vi "DSiam.vi"() -> ()   [LabVIEW 2011]
uses:
  SIAM/SIAM_command.ctl
  SIAM/SIAM-send.ctl
panel:
  out "PWD send":u32[](array[numeric])
  out "code":i32
  out "KEy":string
  out "notifier name":string
  out "send error":errorcluster
  out "value send":dbl
  out "Running":bool
  in  "Scales and Tickets":T1(array[cluster])=[{"ticketID"=514, "Queue/Variable"=FALSE, "name"="stage.z", "Scale"=2e-09, "Offset(HWunits)"=0.0}]
  out "address":string="10.153.70.38"
  out "remote port or service name":u16=3
  out "connect error":errorcluster
  out "Return":i32[](array[numeric]) format="%.0x"
  out "recieve error":errorcluster
  out "Connected":bool
  # "to do\nlimits?\nclosed loop über DSmartmove oder DSIAM oder Smartconnect?\n...\n...\n\n.. Objektivwechsel..."
  # "1122=normal exit"
  # "66=normal exit"
  # "bisher üblich steps/units!!! Logischer für filter!"
  # "becarefull with queues, if there is no reciever it is a memory leak"
  # "ticket  is also inside SIAM-TMSI.vi"
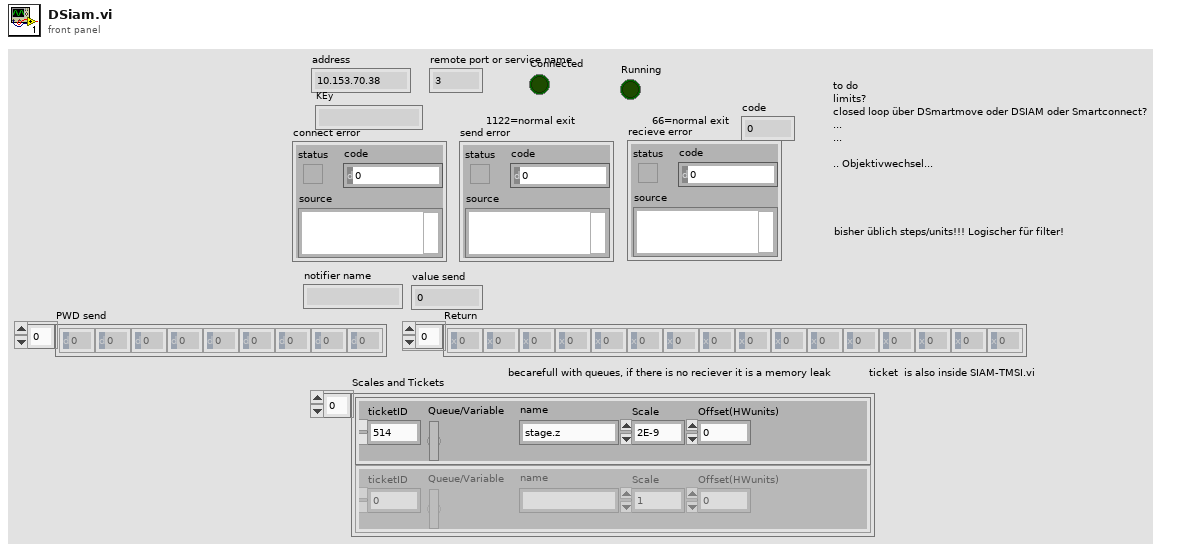
[diagram p1: front panel]
types:
  T1 = cluster{"ticketID":i32, "Queue/Variable":bool, "name":string, "Scale":dbl, "Offset(HWunits)":dbl}[]
  T2 = enum16{"None/#Datasets", "Clear", "TagValueOf#", "AddValues", "ReadValue", "ChangeValue", "Get all"}
  T3 = cluster{"Scale":dbl, "Offset(HWunits)":dbl, "ticketID":i32}[]
  T4 = typedef "SIAM-send.ctl" = enum16{"validID", "storeID", "enable", "rundirect", "sendlist", "run", "stop", "readRegister", "sendValue", "storeStatus"}
  T5 = enum8{"Ch0", "Ch1", "x-Galvo", "y-Galvo", "z-Focus"}
  T6 = enum16{"Ch0", "Ch1", "x-Galvo", "y-Galvo", "z-Focus"}
  T7 = enum16{"Standard", "Buffered", "CRLF", "Immediate"}
  T8 = typedef "SIAM_command.ctl" = u32
  T9 = cluster{"Delay 10µs":u32, "command":T8, "P0":i32, "P1":i32, "P2":i32, "P3":i32, "P4":i32, "P5-ticket":i32}
  T10 = cluster{"Scale":ext, "Offset(HWunits)":ext, "ticketID":i32}[]
  T11 = cluster{"ticketID":i32, "Queue/Variable":bool, "name":string, "Scale":dbl, "Offset(HWunits)":dbl}
  T12 = cluster{"variables":string[], cluster{"Scale":ext, "Offset(HWunits)":ext, "ticketID":i32}[]}
  T13 = cluster{"default value 2":dbl, "default value 1":dbl}
  T14 = cluster{"Delay 10µs":u32, "command":T8, "P0":i32, "P1":i32, "P2":i32, "P3":i32, "P4":i32, "P5-ticket":i32}[]
  T15 = cluster{"Scale":ext, "Offset(HWunits)":ext, "ticketID":i32}
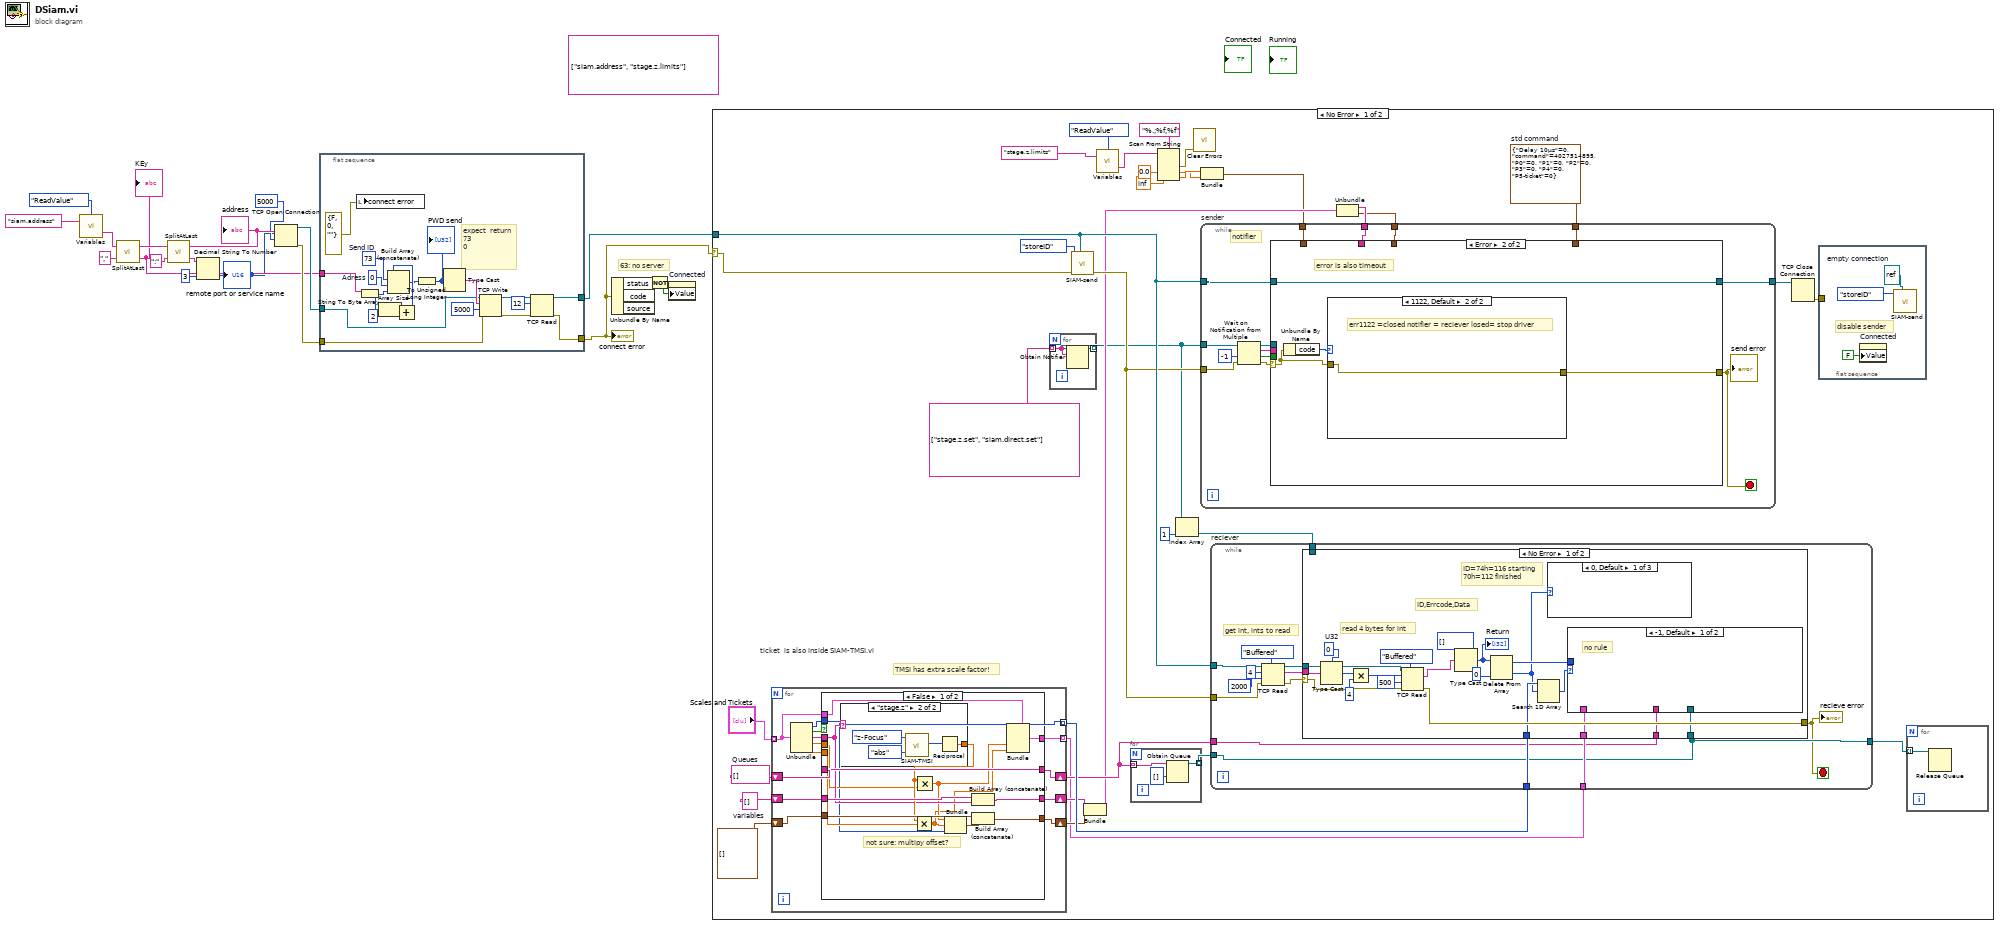
[diagram p0: block diagram]
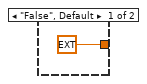
[diagram p2: hidden frame]
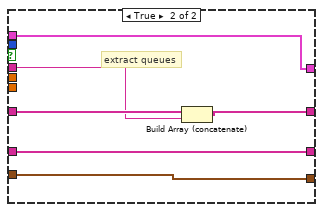
[diagram p3: hidden frame]
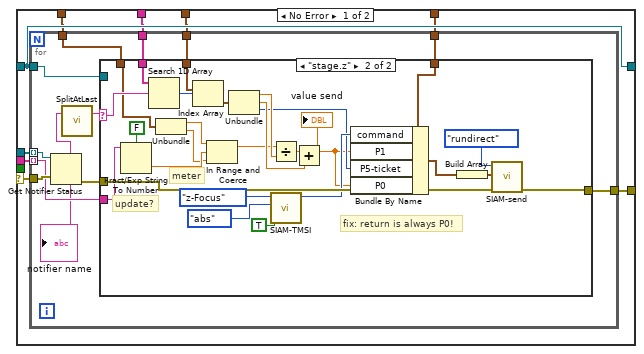
[diagram p4: hidden frame]
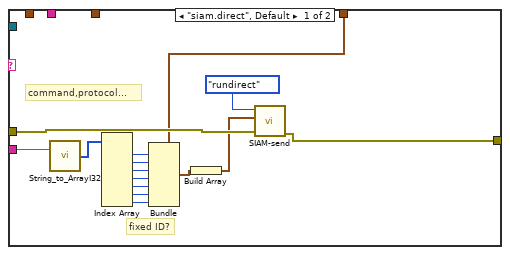
[diagram p5: hidden frame]
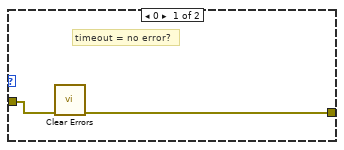
[diagram p6: hidden frame]
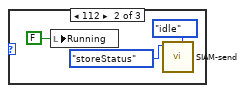
[diagram p7: hidden frame]
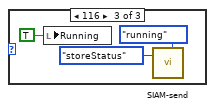
[diagram p8: hidden frame]
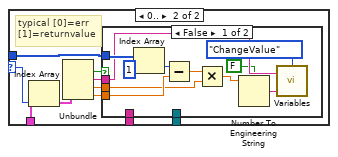
[diagram p9: hidden frame]
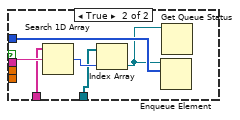
[diagram p10: hidden frame]
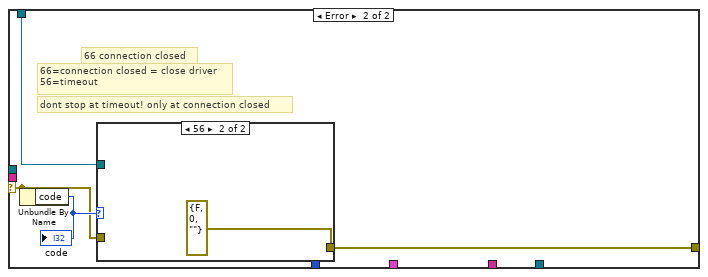
[diagram p11: hidden frame]
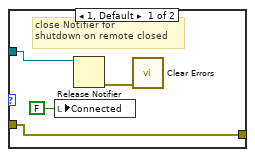
[diagram p12: hidden frame]
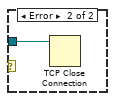
[diagram p13: hidden frame]
diagram:
  (unwired) string[] ["siam.address", "stage.z.limits"]
  # "63: no server"
  n1 = call "Variables.vi"("Tag in"="siam.address", "Command"=T2."ReadValue") -> ("value out"=w9:string)  [unwired: 2 in, 1 out]
  n2 = call "SplitAtLast.vi"("search char"=",", "In-String"=w9) -> ("end"=w4:string, "Front (default)"=w7:string)
  "KEy" <- w4
  n3 = call "SplitAtLast.vi"("search char"=":", "In-String"=w7) -> ("end"=w13:string, "Front (default)"=w14:string)
  "address" <- w14
  n4 = Decimal String To Number(string=w13, default (0L)=3 ("default (0 I32)")) -> (number=w3:i32)  [unwired: 1 in, 1 out]
  "remote port or service name" <- w3
  n5 = TCP Open Connection(address=w14, remote port or service name=w3, timeout ms (60000)=5000) -> (connection ID=w5:refnum<k5>, error out=w6:errorcluster)  [unwired: 1 in, 1 out]
  n6 = flat-sequence {
    tunnel: w5 -> [w33]
    tunnel: w6 -> [w32]
    tunnel: [w22] -> w1
    tunnel: [w24] -> w2
    tunnel: w4 -> [w19]
    frame #0 {
      w30 = 0  # Adress
      w34 = u8 73  # Send ID
      # "expect  return\n73\n0"
      n7 = local write "connect error"(errorcluster {"status"=FALSE, "code"=0, "source"=""} ("recieve error")) -> ()
      n8 = String To Byte Array(string=w19) -> (unsigned byte array=w29:u8[])
      n9 = Array Size(array=w29) -> (size(s)=w35:i32)
      n10 = Add(x=w35, y=2) -> (x+y=w27:i32)
      n11 = Build Array (concatenate)(w27, w34, w30, w29) -> (w26:i32[])
      n12 = To Unsigned Long Integer(number=w26) -> (unsigned 32bit integer=w36:u32[])
      "PWD send" <- w36
      n13 = Type Cast(x=w36) -> (*(type *) &x=w37:string)  [unwired: 1 in]
      n14 = TCP Write(connection ID=w33, data in=w37, error in (no error)=w32, 9:5000 ("timeout ms (25000)")) -> (connection ID out=w25:refnum<k5>, error out=w23:errorcluster)  [unwired: 1 out]
      n15 = TCP Read(connection ID=w25, bytes to read=12, error in (no error)=w23) -> (connection ID out=w24:refnum<k5>, error out=w22:errorcluster)  [unwired: 2 in, 1 out]
    }
  }
  n16 = Unbundle By Name(w1) -> ("status"=w18:bool)  [unwired: 2 out]
  n17 = Not(x=w18) -> (.not. x?=w11:bool)
  n18 = property on="Connected" class="Bool (strict)"("Value"=w11) -> ()  [unwired: 2 in, 2 out]
  n19 = case shown="No Error" w1 {
    selector: w1 -> [w41 _]
    tunnel: w2 -> [w65 w282]
    frame No Error {
      w61 = string[] []  # variables
      w62 = T9 {"Delay 10µs"=0, "command"=4027514895, "P0"=0, "P1"=0, "P2"=0, "P3"=0, "P4"=0, "P5-ticket"=0}  # std command
      w69 = string[] []  # Queues
      # "ticket  is also inside SIAM-TMSI.vi"
      # "TMSI has extra scale factor!"
      n20 = for {
        tunnel: "Scales and Tickets" -> [w86] mode=indexing
        tunnel: [w81] -> w71 mode=indexing
        shift-right: [w91] -> w66
        shift-left: w69 -> [w92]
        shift-right: [w89] -> w59
        shift-left: w61 -> [w90]
        shift-right: [w87] -> w58
        shift-left: T3 [] -> [w88]
        tunnel: [w80] -> w53 mode=indexing
        n21 = Unbundle(w86) -> ("ticketID"=w81:i32, "Queue/Variable"=w85:bool, "name"=w84:string, "Scale"=w83:dbl, "Offset(HWunits)"=w82:dbl)
        n22 = case shown="False" w85 {
          tunnel: w92 -> [w107 w118]
          tunnel: [w107 w116] -> w91
          tunnel: w84 -> [w100 w117]
          tunnel: w86 -> [w96 w113]
          tunnel: w90 -> [w106 w115]
          tunnel: [w105 w115] -> w89
          tunnel: w88 -> [w104 w114]
          tunnel: [w103 w114] -> w87
          tunnel: w83 -> [w98 _]
          tunnel: w82 -> [w99 _]
          tunnel: w81 -> [w97 _]
          tunnel: [w93 w113] -> w80
          frame False {
            # "not sure: multipy offset?"
            n23 = case shown="\"stage.z\"" w100 {
              tunnel: [ext 1.0 w112] -> w101
              frame "False", Default {
              }
              frame "stage.z" {
                n24 = call "SIAM-TMSI.vi"("Type"=enum8{"acc", "vel", "abs", "offset"}."abs", "Motor"=T5."z-Focus") -> ("Resolution-Factor"=w109:i32)  [unwired: 6 in, 3 out]
                n25 = Reciprocal(x=w109) -> (1/x=w112:dbl)
              }
            }
            n26 = Multiply(x=w101, y=w99) -> (x*y=w94:ext)
            n27 = Multiply(x=w101, y=w98) -> (x*y=w95:ext)
            n28 = Bundle(w95, w94, "ticketID"=w97) -> (w102:cluster{ext, ext, "ticketID":i32})  [unwired: 1 in]
            n29 = Build Array (concatenate)(w106, w100) -> (w105:string[])
            n30 = Build Array (concatenate)(w104, w102) -> (w103:T10)
            n31 = Bundle(cluster=w96, "Scale"=w95, "Offset(HWunits)"=w94) -> (w93:T11)  [unwired: 3 in]
          }
          frame True {
            # "extract queues"
            n32 = Build Array (concatenate)(w118, w117) -> (w116:string[])
          }
        }
      }
      n33 = for {
        tunnel: [w120] -> w40 mode=indexing
        tunnel: string[] ["stage.z.set", "siam.direct.set"] -> [w119] mode=indexing
        n34 = Obtain Notifier(name (unnamed)=w119, notification data type=w119) -> (notifier out=w120:refnum<notifier>)  [unwired: 2 in, 2 out]
      }
      n35 = call "SIAM-send.vi"("connection ID"=w65, "error in (no error)"=w41, "command"=SIAM-send."storeID") -> ("error out"=w63:errorcluster)  [unwired: 7 in, 1 out]
      n36 = Bundle("variables"=w59, w58) -> (w57:T12)  [unwired: 1 in]
      n37 = call "Variables.vi"("Tag in"="stage.z.limits", "Command"=T2."ReadValue") -> ("value out"=w50:string)  [unwired: 1 in, 2 out]
      n38 = for {
        tunnel: w66 -> [w79] mode=indexing
        tunnel: [w78] -> w68 mode=indexing
        n39 = Obtain Queue(name (unnamed)=w79, element data type=i32[] []) -> (queue out=w78:refnum<queue>)  [unwired: 3 in, 2 out]
      }
      n40 = Scan From String(format string="%.;%f,%f", input string=w50, default 1=0.0 ("default value 1"), default 2=inf ("default value 2")) -> (error out=w44:errorcluster, output 1=w45:dbl, output 2=w46:dbl)  [unwired: 2 in, 2 out]
      n41 = Index Array(array=w40, index=1) -> (element=w39:refnum<notifier>)
      n42 = call <vilib>:"Clear Errors.vi"("error in (no error)"=w44) -> ()  [unwired: 7 out]
      n43 = Bundle("default value 2"=w46, "default value 1"=w45) -> (w43:T13)  [unwired: 1 out]
      n44 = while "reciever" {
        tunnel: w65 -> [w218]
        tunnel: w71 -> [w211]
        tunnel: w53 -> [w210]
        tunnel: w68 -> [w209]
        tunnel: [w209] -> w67
        tunnel: w66 -> [w208]
        tunnel: w63 -> [w206]
        tunnel: w39 -> [w205]
        stop <- w207 stop-if-true
        # "get int, ints to read"
        n45 = TCP Read(connection ID=w218, bytes to read=4, error in (no error)=w206, 7:T7."Buffered" ("mode (standard)"), 9:2000 ("timeout ms (25000)")) -> (connection ID out=w214:refnum<k5>, data out=w215:string, error out=w212:errorcluster)
        n46 = case shown="No Error" w212 {
          selector: w212 -> [w235 w274]
          tunnel: w215 -> [w239 _]
          tunnel: w214 -> [w236 _]
          tunnel: [w230 w275] -> w207
          tunnel: w211 -> [w225 _]
          tunnel: w210 -> [w224 _]
          tunnel: w209 -> [w220 _]
          tunnel: w208 -> [w219 _]
          tunnel: w205 -> [_ w273]
          frame No Error {
            w238 = u32 0  # U32
            # "ID=74h=116 starting\n70h=112 finished"
            # "read 4 bytes for int"
            # "ID,Errcode,Data"
            n47 = Type Cast(type=w238, x=w239) -> (*(type *) &x=w233:u32)
            n48 = Multiply(x=w233, y=u32 4) -> (x*y=w231:u32)
            n49 = TCP Read(connection ID=w236, bytes to read=w231, error in (no error)=w235, 7:T7."Buffered" ("mode (standard)"), 9:500 ("timeout ms (25000)")) -> (data out=w229:string, error out=w230:errorcluster)  [unwired: 1 out]
            n50 = Type Cast(type=i32[] [], x=w229) -> (*(type *) &x=w227:i32[])
            "Return" <- w227
            n51 = Delete From Array(array=w227, index=0) -> (deleted portion=w221:i32, array with subset deleted=w222:i32[])  [unwired: 1 in]
            n52 = Search 1D Array(1D array=w225, element=w221) -> (index of element=w223:i32)  [unwired: 1 in]
            n53 = case shown="0, Default" w221 {
              frame 0, Default {
              }
              frame 112 {
                n54 = local write "Running"(FALSE ("Running")) -> ()
                n55 = call "SIAM-send.vi"("Value"=enum16{"unknown", "idle", "running", ""}."idle" ("Status"), "command"=SIAM-send."storeStatus") -> ()  [unwired: 8 in, 2 out]
              }
              frame 116 {
                n56 = local write "Running"(TRUE ("Running")) -> ()
                n57 = call "SIAM-send.vi"("Value"=enum16{"unknown", "idle", "running", ""}."running" ("Status"), "command"=SIAM-send."storeStatus") -> ()  [unwired: 8 in, 2 out]
              }
            }
            n58 = case shown="-1, Default" w223 {
              selector: w223 -> [_ w254]
              tunnel: w224 -> [_ w255]
              tunnel: w222 -> [_ w251]
              tunnel: w220 -> [_ w247]
              tunnel: w219 -> [_ w246]
              frame -1, Default {
                # "no rule"
              }
              frame 0.. {
                # "typical [0]=err\n[1]=returnvalue"
                n59 = Index Array(array=w255, index=w254) -> (element=w253:T11)
                n60 = Unbundle(w253) -> ("Queue/Variable"=w252:bool, "name"=w248:string, "Scale"=w249:dbl, "Offset(HWunits)"=w250:dbl)  [unwired: 1 out]
                n61 = case shown="False" w252 {
                  tunnel: w251 -> [w266 w268]
                  tunnel: w250 -> [w264 _]
                  tunnel: w249 -> [w262 _]
                  tunnel: w248 -> [w261 w272]
                  tunnel: w247 -> [_ w269]
                  tunnel: w246 -> [_ w271]
                  frame False {
                    n62 = Index Array(array=w266, index=1) -> (element=w265:i32)
                    n63 = Subtract(x=w265, y=w264) -> (x-y=w263:dbl)
                    n64 = Multiply(x=w263, y=w262) -> (x*y=w259:dbl)
                    n65 = Number To Engineering String(1:FALSE ("use system decimal point (T)"), 4:w259) -> (0:w258:string)  [unwired: 2 out]
                    n66 = call "Variables.vi"("value"=w258, "Tag in"=w261, "Command"=T2."ChangeValue") -> ()  [unwired: 1 in, 2 out]
                  }
                  frame True {
                    n67 = Search 1D Array(1D array=w271, element=w272) -> (index of element=w270:i32)  [unwired: 1 in]
                    n68 = Index Array(array=w269, index=w270) -> (element=w267:refnum<queue>)
                    n69 = Enqueue Element(queue=w267, element=w268) -> ()  [unwired: 2 in, 3 out]
                    n70 = Get Queue Status(queue=w267) -> ()  [unwired: 2 in, 8 out]
                  }
                }
              }
            }
          }
          frame Error {
            # "66 connection closed"
            # "dont stop at timeout! only at connection closed"
            # "66=connection closed = close driver\n56=timeout"
            n71 = Unbundle By Name(w274) -> ("code"=w276:i32)
            "code" <- w276
            n72 = case shown="56" w276 {
              tunnel: [w280 errorcluster {"status"=FALSE, "code"=0, "source"=""} ("error out")] -> w275
              tunnel: w274 -> [w280 _]
              tunnel: w273 -> [w278 _]
              frame 1, Default {
                # "close Notifier for\nshutdown on remote closed"
                n73 = local write "Connected"(FALSE ("Connected")) -> ()
                n74 = Release Notifier(notifier=w278) -> (error out=w277:errorcluster)  [unwired: 2 in, 2 out]
                n75 = call <vilib>:"Clear Errors.vi"("error in (no error)"=w277) -> ()  [unwired: 6 in, 1 out]
              }
              frame 56 {
              }
            }
          }
        }
        "recieve error" <- w207
      }
      n76 = Unbundle(w57) -> ("variables"=w56:string[], w55:T10)
      n77 = while "sender" {
        tunnel: w65 -> [w132]
        tunnel: w40 -> [w131]
        tunnel: [w129] -> w70
        tunnel: w63 -> [w128]
        tunnel: w62 -> [w124]
        tunnel: w56 -> [w123]
        tunnel: w55 -> [w122]
        tunnel: w43 -> [w121]
        stop <- w125 stop-if-true
        # "notifier"
        n78 = Wait on Notification from Multiple(0:w131, 2:-1 ("timeout in ms (-1)"), 3:w128) -> (8:w134:refnum<notifier>[], 9:w133:string[], 10:w126:bool, 11:w127:errorcluster)  [unwired: 1 in]
        n79 = case shown="Error" w127 {
          selector: w127 -> [w140 w198]
          tunnel: w134 -> [w143 _]
          tunnel: w133 -> [w142 _]
          tunnel: w132 -> [w141 w201]
          tunnel: [w141 w201] -> w129
          tunnel: w126 -> [_ _]
          tunnel: [w139 w200] -> w125
          tunnel: w124 -> [w138 _]
          tunnel: w123 -> [w137 _]
          tunnel: w122 -> [w136 _]
          tunnel: w121 -> [w135 _]
          frame No Error {
            n80 = for {
              tunnel: w143 -> [w154] mode=indexing
              tunnel: w142 -> [w153] mode=indexing
              tunnel: w141 -> [w152]
              tunnel: w140 -> [w155]
              tunnel: [w151] -> w139
              tunnel: w138 -> [w149]
              tunnel: w137 -> [w148]
              tunnel: w136 -> [w147]
              tunnel: w135 -> [w144]
              n81 = Get Notifier Status(notifier=w154, error in (no error)=w155) -> (notifier name=w146:string, error out=w150:errorcluster)  [unwired: 3 out]
              "notifier name" <- w146
              n82 = call "SplitAtLast.vi"("In-String"=w146) -> ("Front (default)"=w145:string)  [unwired: 1 in, 1 out]
              n83 = case shown="\"stage.z\"" w145 {
                selector: w145 -> [_ w192]
                tunnel: w153 -> [w167 w196]
                tunnel: w152 -> [_ _]
                tunnel: [w169 w178] -> w151
                tunnel: w150 -> [w168 w197]
                tunnel: w149 -> [w165 w186]
                tunnel: w148 -> [_ w191]
                tunnel: w147 -> [_ w189]
                tunnel: w144 -> [_ w173]
                frame "siam.direct", Default {
                  # "fixed ID?"
                  # "command,protocol..."
                  n84 = call "String_to_ArrayI32.vi"("String"=w167) -> ("ArrayI32"=w166:i32[])  [unwired: 1 in]
                  n85 = Index Array(array=w166) -> (element #1=w164:i32, element #2=w163:i32, element #3=w162:i32, element #4=w161:i32, element #5=w160:i32, element #6=w159:i32, element #7=w158:i32)  [unwired: 7 in]
                  n86 = Bundle(cluster=w165, "command"=w164, "P0"=w163, "P1"=w162, "P2"=w161, "P3"=w160, "P4"=w159, "P5-ticket"=w158) -> (w157:T9)  [unwired: 1 in]
                  n87 = Build Array(w157) -> (w156:T14)
                  n88 = call "SIAM-send.vi"("error in (no error)"=w168, "Script"=w156, "command"=SIAM-send."rundirect") -> ("error out"=w169:errorcluster)  [unwired: 7 in, 1 out]
                }
                frame "stage.z" {
                  # "fix: return is always P0!"
                  # "meter"
                  # "update?"
                  n89 = Fract/Exp String To Number(use system decimal point (T)=FALSE, string=w196) -> (number=w176:dbl)  [unwired: 2 in, 1 out]
                  n90 = Search 1D Array(1D array=w191, element=w192) -> (index of element=w190:i32)  [unwired: 1 in]
                  n91 = Unbundle(w173) -> ("default value 2"=w174:dbl, "default value 1"=w175:dbl)
                  n92 = Index Array(array=w189, index=w190) -> (element=w188:T15)
                  n93 = In Range and Coerce(upper limit=w174, x=w176, lower limit=w175) -> (coerced(x)=w172:dbl)  [unwired: 1 out]
                  n94 = Unbundle(w188) -> ("Scale"=w184:ext, "Offset(HWunits)"=w183:ext, "ticketID"=w177:i32)
                  n95 = Divide(x=w172, y=w184) -> (x/y=w187:ext)
                  n96 = call "SIAM-TMSI.vi"("use ticket"=TRUE, "Type"=enum8{"acc", "vel", "abs", "offset"}."abs", "Motor"=T6."z-Focus") -> ("command"=w180:T8)  [unwired: 5 in, 3 out]
                  n97 = Add(x=w187, y=w183) -> (x+y=w171:ext)
                  "value send" <- w171
                  n98 = Bundle By Name(cluster=w186, "command"=w180, "P1"=w171, "P5-ticket"=w177, "P0"=w171) -> (w194:T9)
                  n99 = Build Array(w194) -> (w193:T14)
                  n100 = call "SIAM-send.vi"("error in (no error)"=w197, "Script"=w193, "command"=SIAM-send."rundirect") -> ("error out"=w178:errorcluster)  [unwired: 7 in, 1 out]
                }
              }
            }
          }
          frame Error {
            # "error is also timeout"
            n101 = Unbundle By Name(w198) -> ("code"=w199:i32)
            n102 = case shown="1122, Default" w199 {
              tunnel: [w203 w204] -> w200
              tunnel: w198 -> [w202 w204]
              frame 0 {
                # "timeout = no error?"
                n103 = call <vilib>:"Clear Errors.vi"("error in (no error)"=w202) -> ("error out"=w203:errorcluster)  [unwired: 6 in]
              }
              frame 1122, Default {
                # "err1122 =closed notifier = reciever losed= stop driver"
              }
            }
          }
        }
        "send error" <- w125
      }
      n104 = TCP Close Connection(connection ID=w70) -> (error out=w42:errorcluster)  [unwired: 2 in, 1 out]
      n105 = flat-sequence {
        tunnel: w42 -> [_]
        frame #0 {
          w74 = refnum<k5> refnum  # empty connection
          # "disable sender"
          n106 = property on="Connected" class="Bool (strict)"("Value"=FALSE ("Connected")) -> ()  [unwired: 2 in, 2 out]
          n107 = call "SIAM-send.vi"("connection ID"=w74, "command"=SIAM-send."storeID") -> ()  [unwired: 8 in, 2 out]
        }
      }
      n108 = for {
        tunnel: w67 -> [w76] mode=indexing
        n109 = Release Queue(queue=w76) -> ()  [unwired: 2 in, 3 out]
      }
    }
    frame Error {
      n110 = TCP Close Connection(connection ID=w282) -> ()  [unwired: 2 in, 2 out]
    }
  }
  "connect error" <- w1
